vi "OPC Main.vi"(7 "Name of Parent Panel":string="Main.vi", 9 "New Center Coords":T2={"Horizontal"=470, "Vertical"=200}, 10 "Config":variant, 11 "Main UI Message Queue":refnum<queue>) -> ()   [LabVIEW 2018, in "OPC UA.lvlib"]
uses:
  OPC UA.lvlib
  support/Message Queue/Message Cluster.ctl
  <vilib>/Utility/miscctls.llb/LVPoint32TypeDef.ctl
  OPC Tag Data.ctl
  controls/UI State.ctl
  OPC Module Config.ctl
  Scale Module Folder/Measure Instrument/State Enum.ctl
  OPC Settings.ctl
  Variable Data Cluster.ctl
  <vilib>/OPCUA/controls/NodeId.ctl
  <vilib>/OPCUA/controls/OPC UA StatusCode.ctl
  <vilib>/OPCUA/controls/Subscription ID.ctl
  <vilib>/OPCUA/controls/OPC UA Client Refnum.ctl
  <vilib>/OPCUA/controls/Subscription Data Change.ctl
  <vilib>/OPCUA/controls/Data Type.ctl
  OPC Display Cluster.ctl
  support/Message Queue/Enqueue Message (Single).vi
  support/Message Queue/Message Queue.lvlib
  support/Support Library.lvlib
  support/Command Log VIs/Command Logging.lvlib
  support/User Event - Stop/User Event - Stop.lvlib
  OPC Dialog.vi
  Scale Module Folder/Measure Instrument/Scale Module Engine.lvlib
  OPC UA Module Engine.lvlib
  Report Generation/Report Generation.lvlib
panel:
  out "Tag Data 2":T1[](array[typedef])
  out "Configuration.server endpoint URL":string
  out "Updating":bool
  out "ScanCode":i16
  in  "Settings Button":bool
  in  "Exit":bool
  out "Status":string
  out "Log File path":path
  out "server endpoint URL":string
  # "opc.tcp://localhost:49580"
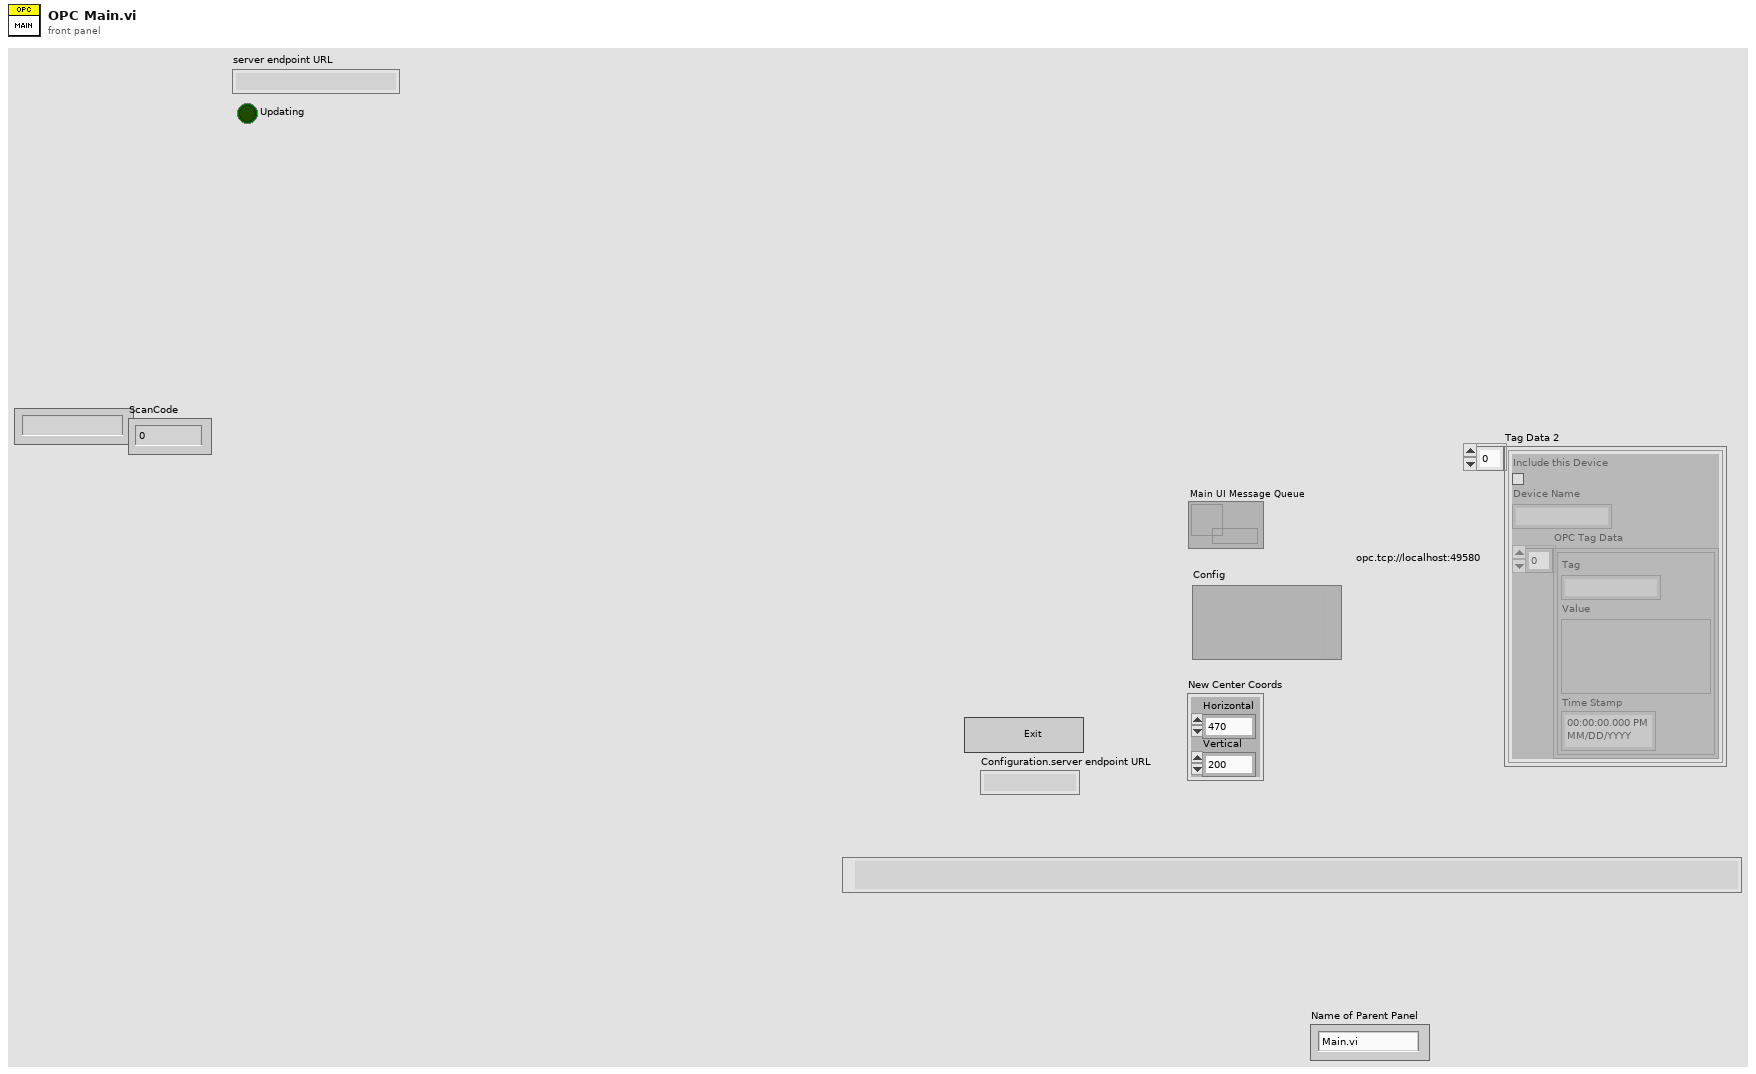
[diagram p1: front panel]
types:
  T1 = typedef "OPC UA.lvlib/OPC Tag Data.ctl" = cluster{"Include this Device":bool, "Device Name":string, "OPC Tag Data":cluster{"Tag":string, "Value":variant, "Time Stamp":timestamp}[]}
  T2 = typedef "LVPoint32TypeDef.ctl" = cluster{"Horizontal":i32, "Vertical":i32}
  T3 = enum32{"Invalid", "Default", "Floating", "Floating/Auto-Hide", "Modal"}
  T4 = typedef "OPC UA.lvlib/OPC Module Config.ctl" = cluster{"State":T5, "GUID":string, "Process Name":string, "User name":string, "Drop Coords":T2, "Configuration":T6, "First Iteration":bool, "Data":cluster{"Object Name":string, "Variable Array":T7[]}[], "Load Count":i32, "Log Started":bool, "subscription ID out":T10, "OPC UA client refnum out":T11, "Event Registration Refnum":refnum<event-registration>, "Start Time":timestamp, "Current Time":timestamp, "Tag Data":T1[]}
  T5 = typedef "Scale Module.lvlib/Scale Module Engine.lvlib/State Enum.ctl" = enum16{"Measuring", "Idle"}
  T6 = typedef "OPC UA.lvlib/OPC Settings.ctl" = cluster{"Cycle Period":dbl, "server endpoint URL":string, "security policy":cluster{"message mode":enum16{"None", "Sign", "Sign and Encrypt"}, "security":enum16{"Basic256", "Basic128Rsa15"}}, "Trust Any Server":bool}
  T7 = typedef "OPC UA.lvlib/Variable Data Cluster.ctl" = cluster{"node ID":T8, "browse name":string, "status":T9, "timestamp":timestamp, "value ":variant}
  T8 = typedef "NodeId.ctl" = string
  T9 = typedef "OPC UA StatusCode.ctl" = u32
  T10 = typedef "Subscription ID.ctl" = u32
  T11 = typedef "OPC UA Client Refnum.ctl" = refnum<k21>
  T12 = typedef "UI State.ctl" = enum16{"Idle", "Acquiring and Logging", "Waiting for Exit", "Waiting for Exit (Acq Stopped)", "Waiting for Exit (Log Stopped)", "Waiting for Stop", "Waiting for Stop (Acq Stopped)", "Waiting for Stop (Log Stopped)"}
  T13 = typedef "OPC UA.lvlib/Message Queues.ctl" = cluster{"OPC UI":refnum<queue>, "OPC Engine":refnum<queue>, "OPC Display":refnum<queue>}
  T14 = typedef "OPC UA.lvlib/OPC Display Cluster.ctl" = cluster{"URL":string, "Cycle":i32, "Updating":bool, "Tag Data":T1[]}
  T15 = cluster{"Shift":bool, "Ctrl":bool, "Alt":bool, "Cmd":bool, "Opt":bool}
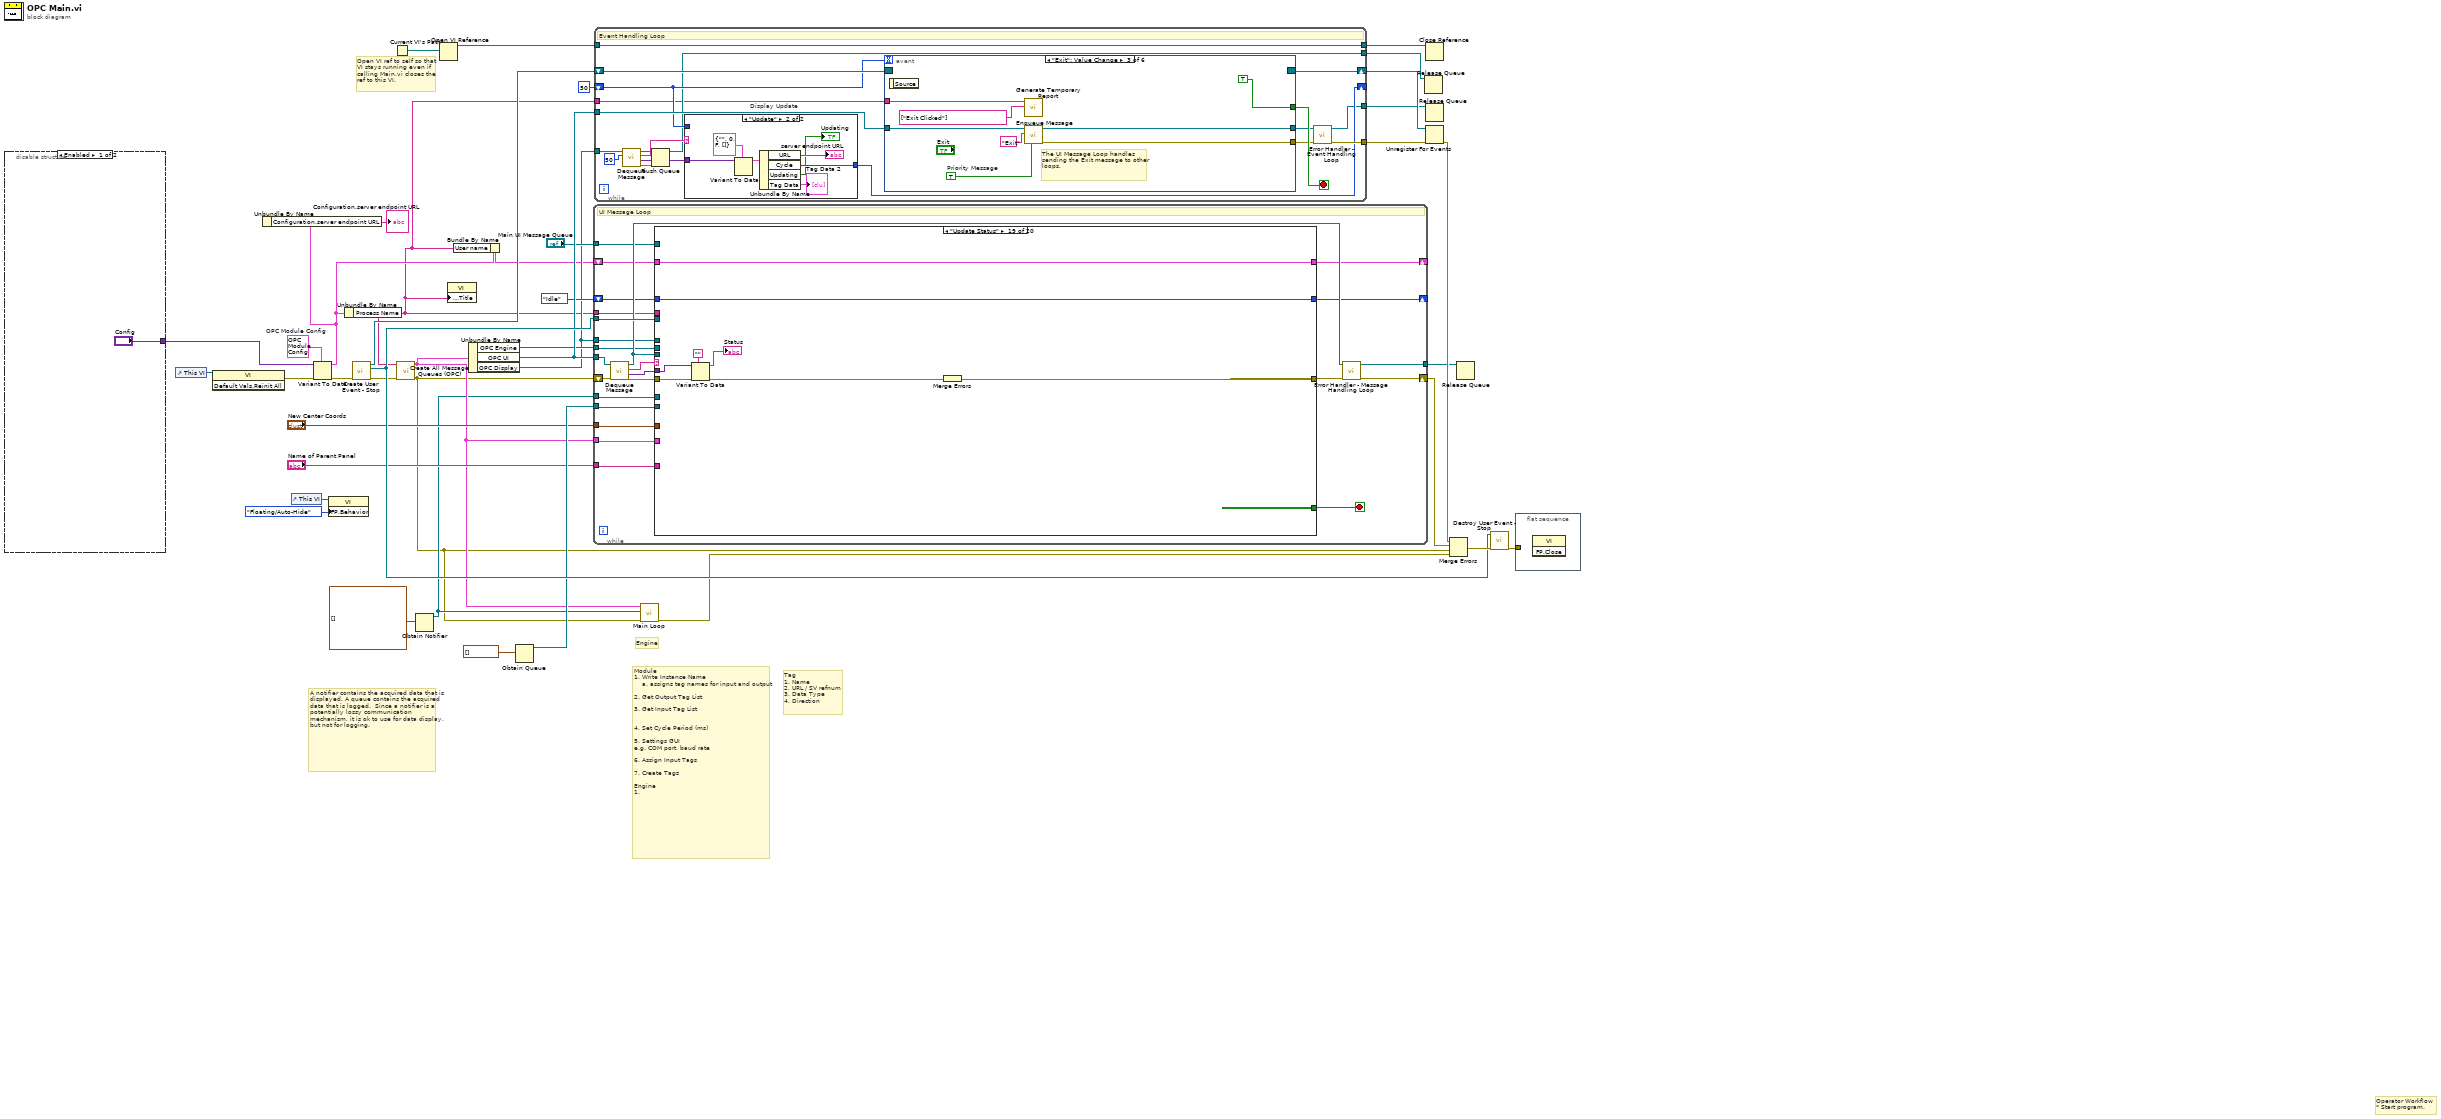
[diagram p0: block diagram]
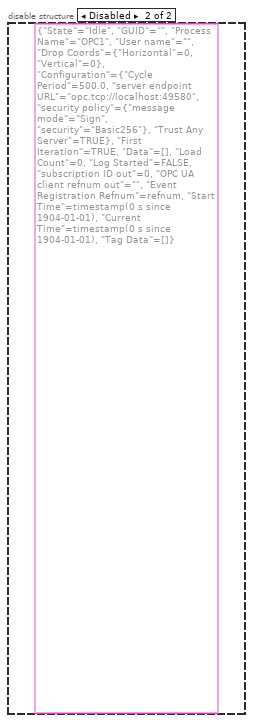
[diagram p2: hidden frame]
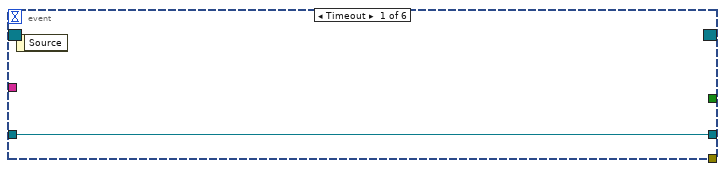
[diagram p4: hidden frame]
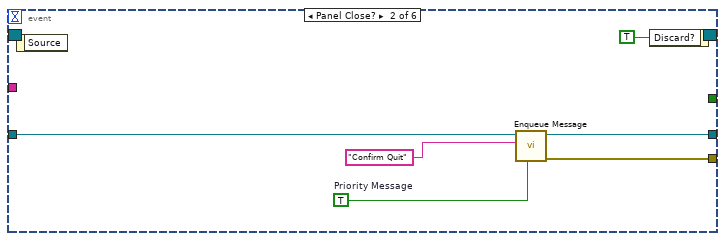
[diagram p5: hidden frame]
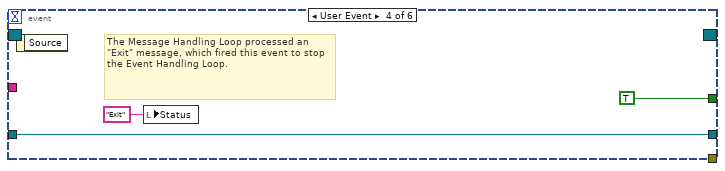
[diagram p6: hidden frame]
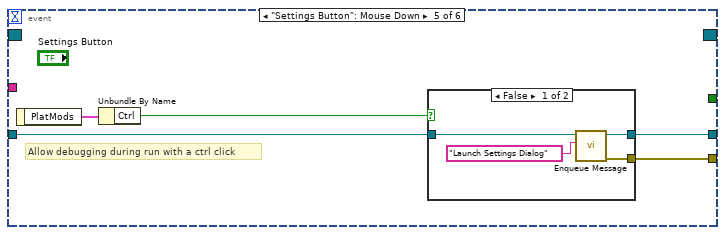
[diagram p7: hidden frame]
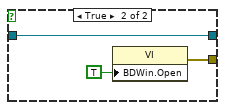
[diagram p8: hidden frame]
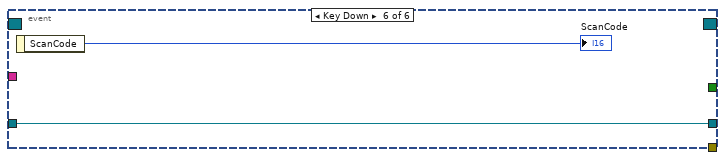
[diagram p9: hidden frame]
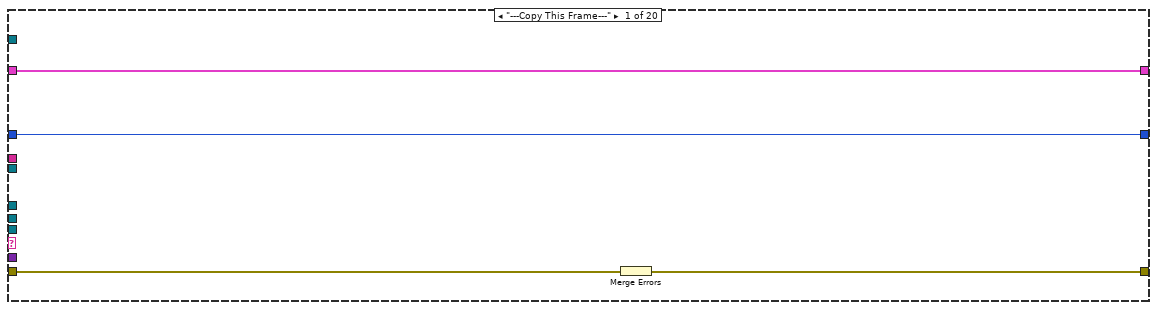
[diagram p10: hidden frame]
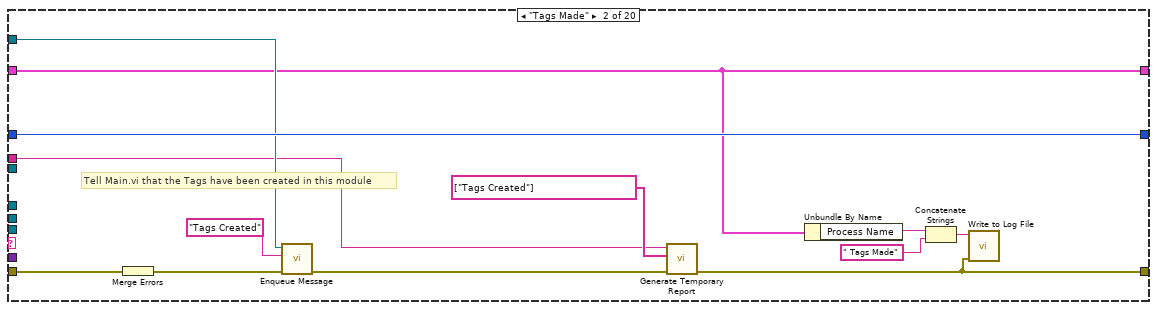
[diagram p11: hidden frame]
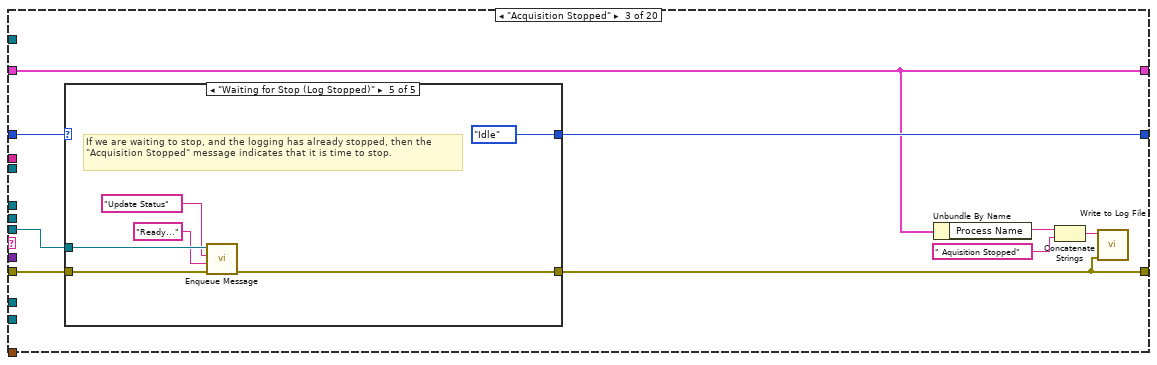
[diagram p12: hidden frame]
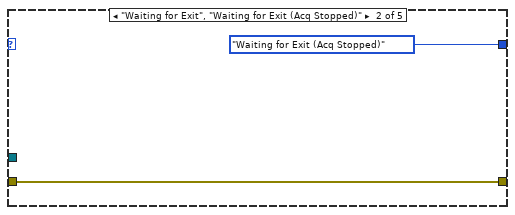
[diagram p14: hidden frame]
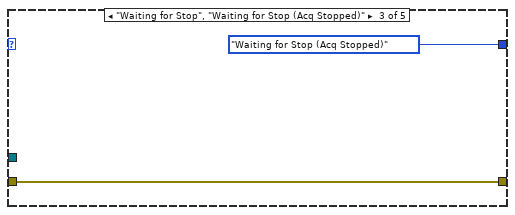
[diagram p15: hidden frame]
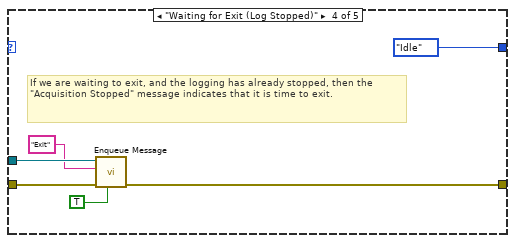
[diagram p16: hidden frame]
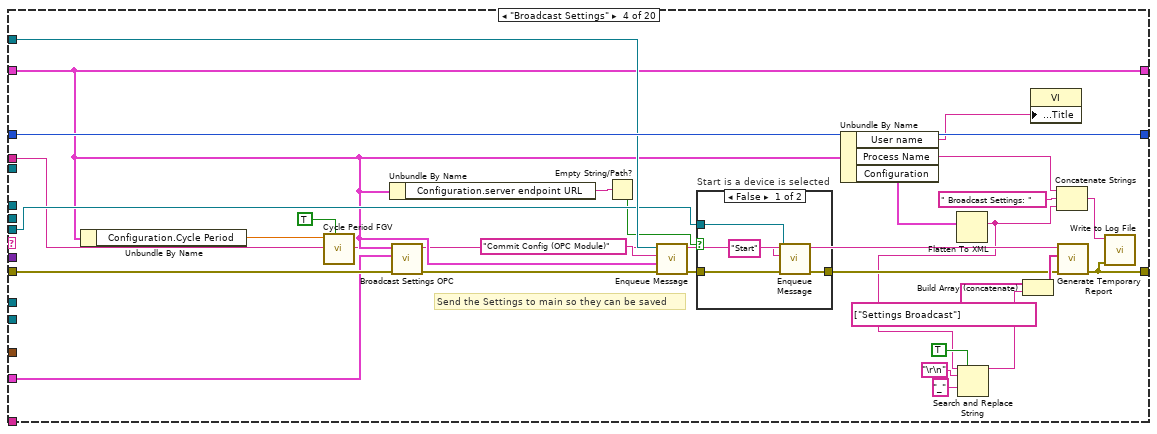
[diagram p17: hidden frame]
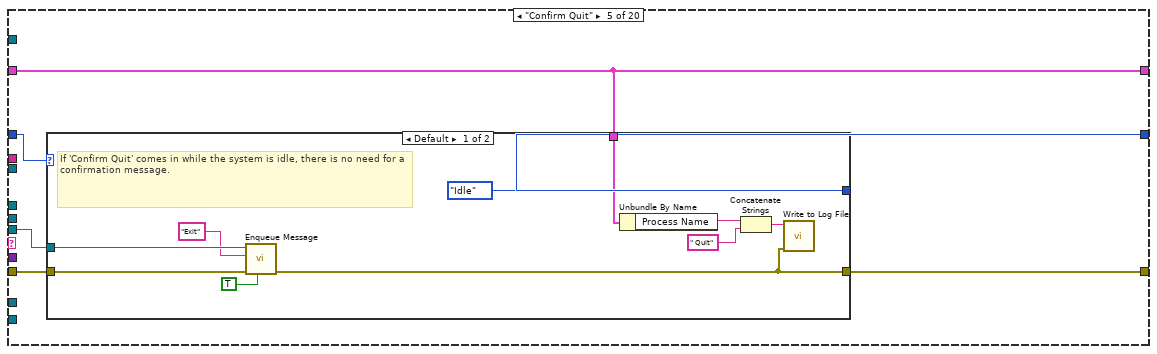
[diagram p19: hidden frame]
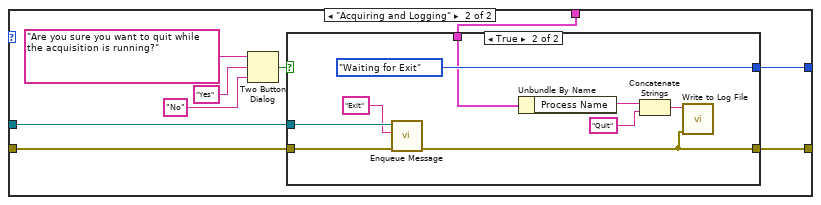
[diagram p20: hidden frame]
diagram:
  w7 = T4 {"State"=enum."Idle", "GUID"="", "Process Name"="", "User name"="", "Drop Coords"={"Horizontal"=0, "Vertical"=0}, "Configuration"={"Cycle Period"=500.0, "server endpoint URL"="", "security policy"={"message mode"=enum."Sign", "security"=enum."Basic256"}, "Trust Any Server"=FALSE}, "First Iteration"=FALSE, "Data"=[], "Load Count"=0, "Log Started"=FALSE, "subscription ID out"=0, "OPC UA client refnum out"="", "Event Registration Refnum"=refnum, "Start Time"=timestamp(0 s since 1904-01-01), "Current Time"=timestamp(0 s since 1904-01-01), "Tag Data"=[]}  # OPC Module Config
  # "Open VI ref to self so that\nVI stays running even if\ncalling Main.vi closes the\nref to this VI."
  # "Engine"
  # "Operator Workflow\n* Start program."
  # "Module \n1. Write Instance Name\n    a. assigns tag names for input and output\n\n2. Get Output Tag List\n\n3. Get Input Tag List\n\n\n4. Set Cycle Period (ms)\n\n5. Settings GUI\ne.g. COM port, baud rate\n\n6. Assign Input Tags\n\n7. Create Tags\n\nEngine\n1."
  # "Tag\n1. Name\n2. URL / SV refnum\n3. Data Type\n4. Direction"
  # "A notifier contains the acquired data that is displayed. A queue contains the acquired data that is logged.  Since a notifier is a potentially lossy communication mechanism, it is ok to use for data display, but not for logging."
  n1 = disable-structure shown="Enabled" {
    disable-tunnel: ["Config" _] -> w14
    frame Enabled {
    }
    frame Disabled {
      (unwired) T4 {"State"=enum."Idle", "GUID"="", "Process Name"="OPC1", "User name"="", "Drop Coords"={"Horizontal"=0, "Vertical"=0}, "Configuration"={"Cycle Period"=500.0, "server endpoint URL"="opc.tcp://localhost:49580", "security policy"={"message mode"=enum."Sign", "security"=enum."Basic256"}, "Trust Any Server"=TRUE}, "First Iteration"=TRUE, "Data"=[], "Load Count"=0, "Log Started"=FALSE, "subscription ID out"=0, "OPC UA client refnum out"="", "Event Registration Refnum"=refnum, "Start Time"=timestamp(0 s since 1904-01-01), "Current Time"=timestamp(0 s since 1904-01-01), "Tag Data"=[]} ("OPC Module Config")
    }
  }
  n2 = control-ref of="This VI"() -> (w6:refnum<vi>)
  n3 = invoke class="VI" method="Default Vals.Reinit All"(reference=w6) -> (error out=w20:errorcluster)  [unwired: 2 in, 2 out]
  n4 = control-ref of="This VI"() -> (w5:refnum<vi>)
  n5 = Variant To Data(error in=w20, type=w7, Variant=w14) -> (data=w3:T4, error out=w25:errorcluster)
  n6 = Unbundle By Name(w3) -> ("Configuration.server endpoint URL"=→"Configuration.server endpoint URL":string)
  n7 = property class="VI"(reference=w5, "FP.Behavior"=T3."Floating/Auto-Hide" ("Front Panel Window:Behavior")) -> ()  [unwired: 1 in, 2 out]
  n8 = Unbundle By Name(w3) -> ("Process Name"=w1:string)
  n9 = call "Create User Event - Stop.vi"("error in (no error)"=w25) -> ("error out"=w19:errorcluster, "User Event - Stop"=w37:refnum<user-event>, "Stop Event Registration Refnum"=w38:refnum<event-registration>)  [unwired: 8 in]
  n10 = Current VI's Path() -> (path=w26:path)
  n11 = call "Create All Message Queues (OPC).vi"("error in (no error)"=w19, "Process Name"=w1) -> ("error out"=w16:errorcluster, "Message Queues"=w18:T13)  [unwired: 8 in]
  n12 = Obtain Notifier(notification data type=waveform(dbl)[] []) -> (notifier out=w17:refnum<notifier>)  [unwired: 3 in, 2 out]
  n13 = Open VI Reference(vi path=w26) -> (vi reference=w27:refnum<vi>)  [unwired: 5 in, 1 out]
  n14 = property class="VI"("Front Panel.Title"=w1) -> ()  [unwired: 2 in, 2 out]
  n15 = Bundle By Name(cluster=w3, "User name"=w1) -> (w2:T4)
  n16 = Unbundle By Name(w18) -> ("OPC Engine"=w30:refnum<queue>, "OPC UI"=w34:refnum<queue>, "OPC Display"=w13:refnum<queue>)
  n17 = Obtain Queue(element data type=waveform(dbl)[] []) -> (queue out=w29:refnum<queue>)  [unwired: 4 in, 2 out]
  n18 = while {
    tunnel: w34 -> [w61]
    tunnel: w37 -> [w65]
    shift-right: [w57] -> w41
    shift-left: w16 -> [w64]
    shift-right: [w43] -> _
    shift-left: w2 -> [w50]
    tunnel: w17 -> [w60]
    tunnel: w29 -> [w59]
    shift-right: [w54] -> _
    shift-left: UI_State."Idle" ("UI State") -> [w55]
    tunnel: w30 -> [w53]
    tunnel: w18 -> [w52]
    tunnel: "Main UI Message Queue" -> [w49]
    tunnel: w1 -> [w48]
    tunnel: "New Center Coords" -> [w47]
    tunnel: "Name of Parent Panel" -> [w46]
    tunnel: w13 -> [w45]
    tunnel: [w44] -> w8
    stop <- w66 stop-if-true
    # "UI Message Loop"
    n19 = call "Dequeue Message.vi"("error in (no error)"=w64, "Message Queue"=w61) -> ("error out"=w51:errorcluster, "Message Data"=w62:variant, "Message"=w63:string, "dup Message Queue"=w56:refnum<queue>)  [unwired: 6 in]
    n20 = case "Message Cases" shown="\"Update Status\"" w63 {
      selector: w63 -> [_ _ _ _ _ _ _ _ _ _ _ _ _ _ _ _ _ _ _ w417]
      tunnel: w56 -> [_ _ w89 w133 w148 _ w201 w215 w239 _ w281 w298 w314 _ w352 _ _ w405 _ _]
      tunnel: w51 -> [w70 w83 w90 w126 w147 w182 w196 w219 w238 w264 w277 w293 w315 w338 w351 w360 w372 w400 w414 _]
      tunnel: [w69 w71 w85 w116 w146 w183 w188 w206 w221 w264 w265 w288 w310 w341 w346 w357 w374 w388 w415 w416] -> w58
      tunnel: [_ _ _ _ _ _ _ _ TRUE _ _ _ _ _ _ _ _ _ _ _] -> w66
      tunnel: w62 -> [_ _ _ _ _ w185 _ w218 w228 _ _ _ _ w339 _ _ _ _ w413 _]
      tunnel: w65 -> [_ _ _ _ _ _ _ _ w249 _ _ _ _ _ _ _ _ _ _ _]
      tunnel: w50 -> [w67 w75 w84 w123 w144 w180 w191 w205 w224 w261 w269 w291 w309 w345 w347 w361 w373 w392 w408 w422]
      tunnel: w60 -> [_ _ _ _ _ _ _ _ w247 _ _ _ _ _ _ _ _ _ _ _]
      tunnel: w59 -> [_ _ _ _ _ _ _ _ w243 _ _ _ _ _ _ _ _ _ _ _]
      tunnel: w55 -> [w68 w82 w92 w138 w149 w181 w197 w210 w236 _ _ w300 w317 w344 _ _ _ w401 w409 w426]
      tunnel: [w68 w82 w91 w138 w145 w181 w198 w210 w235 UI_State."Idle" ("UI State") UI_State."Idle" ("UI State") w300 w316 w344 UI_State."Acquiring and Logging" ("UI State") UI_State."Acquiring and Logging" ("UI State") UI_State."Acquiring and Logging" ("UI State") w402 w409 w426] -> w54
      tunnel: w53 -> [_ _ _ _ _ _ _ _ w242 _ _ _ _ _ _ w365 w381 w399 _ _]
      tunnel: w52 -> [_ _ _ w124 _ _ _ _ _ _ _ _ _ _ _ _ _ _ _ _]
      tunnel: w49 -> [_ w79 _ w134 _ _ _ _ w227 _ _ w299 _ _ _ _ _ _ _ _]
      tunnel: [w67 w75 w84 w123 w144 w180 w191 w205 w224 w261 w269 w292 w309 w345 w347 w361 w373 w392 w408 w422] -> w43
      tunnel: w48 -> [_ w73 _ w118 _ _ w187 _ _ _ w275 _ _ _ _ w356 _ w390 _ _]
      tunnel: w47 -> [_ _ _ _ _ _ _ _ _ _ w274 _ _ _ _ _ _ _ _ _]
      tunnel: w46 -> [_ _ _ _ _ _ _ _ _ _ w273 _ _ _ _ _ _ _ _ _]
      tunnel: w45 -> [_ _ _ _ _ _ _ _ _ _ w268 _ _ _ _ _ _ _ _ _]
      frame "---Copy This Frame---" {
        # "Duplicate this frame when creating new messages.  Change this comment in the duplicated frame to describe this message."
        n21 = Merge Errors(w70) -> (w69:errorcluster)
      }
      frame "Tags Made" {
        # "Tell Main.vi that the Tags have been created in this module"
        # "Duplicate this frame when creating new messages.  Change this comment in the duplicated frame to describe this message."
        n22 = Merge Errors(w83) -> (w80:errorcluster)
        n23 = call-poly "Enqueue Message.vi"("error in (no error)"=w80, "Message"="Tags Created", "Message Queue"=w79) -> ("error out"=w72:errorcluster)  [unwired: 7 in, 1 out]
        n24 = call "Generate Temporary Report.vi"("error in (no error)"=w72, "Line of Events"=string[] ["Tags Created"], "Module Name"=w73) -> ("error out"=w71:errorcluster)  [unwired: 8 in]
        n25 = Unbundle By Name(w75) -> ("Process Name"=w78:string)
        n26 = Concatenate Strings(w78, " Tags Made" ("text")) -> (w76:string)
        n27 = call "Write to Log File.vi"("error in"=w71, "text"=w76) -> ()  [unwired: 9 in, 1 out]
      }
      frame "Acquisition Stopped" {
        # "Logic for determining what action to take when the acquisition has stopped."
        n28 = case shown="\"Waiting for Stop (Log Stopped)\"" w92 {
          selector: w92 -> [w94 _ _ _ _]
          tunnel: [w94 UI_State."Waiting for Exit (Acq Stopped)" ("UI State") UI_State."Waiting for Stop (Acq Stopped)" ("UI State") UI_State."Idle" ("UI State") UI_State."Idle" ("UI State")] -> w91
          tunnel: w90 -> [w93 w95 w97 w103 w109]
          tunnel: [w93 w95 w97 w102 w108] -> w85
          tunnel: w89 -> [_ _ _ w101 w107]
          frame Default {
          }
          frame "Waiting for Exit", "Waiting for Exit (Acq Stopped)" {
          }
          frame "Waiting for Stop", "Waiting for Stop (Acq Stopped)" {
          }
          frame "Waiting for Exit (Log Stopped)" {
            # "If we are waiting to exit, and the logging has already stopped, then the \"Acquisition Stopped\" message indicates that it is time to exit."
            n29 = call-poly "Enqueue Message.vi"("Priority Message? (F)"=TRUE, "error in (no error)"=w103, "Message"="Exit", "Message Queue"=w101) -> ("error out"=w102:errorcluster)  [unwired: 6 in, 1 out]
          }
          frame "Waiting for Stop (Log Stopped)" {
            # "If we are waiting to stop, and the logging has already stopped, then the \"Acquisition Stopped\" message indicates that it is time to stop."
            n30 = call-poly "Enqueue Message.vi"("error in (no error)"=w109, "Message Data"="Ready..." ("Message"), "Message"="Update Status", "Message Queue"=w107) -> ("error out"=w108:errorcluster)  [unwired: 6 in, 1 out]
          }
        }
        n31 = Unbundle By Name(w84) -> ("Process Name"=w88:string)
        n32 = Concatenate Strings(w88, " Aquisition Stopped" ("text")) -> (w86:string)
        n33 = call "Write to Log File.vi"("error in"=w85, "text"=w86) -> ()  [unwired: 9 in, 1 out]
      }
      frame "Broadcast Settings" {
        # "Send the Settings to main so they can be saved"
        # "Send the 'Update Settings' message to the Logging and Acquisition message loops."
        n34 = Unbundle By Name(w123) -> ("Configuration.Cycle Period"=w136:dbl)
        n35 = call "Cycle Period FGV.vi"("Write"=TRUE, "Cycle Period In (ms)"=w136) -> ()  [unwired: 8 in, 2 out]
        n36 = Unbundle By Name(w123) -> ("Configuration.server endpoint URL"=w128:string)
        n37 = call "Broadcast Settings OPC.vi"("error in (no error)"=w126, "Message Queues"=w124, "OPC Module Config"=w123) -> ("error out"=w125:errorcluster)  [unwired: 8 in]
        n38 = Empty String/Path?(string/path=w128) -> (empty?=w127:bool)
        n39 = call-poly "Enqueue Message.vi"("error in (no error)"=w125, "Message Data"=w123, "Message"="Commit Config (OPC Module)", "Message Queue"=w134) -> ("error out"=w132:errorcluster)  [unwired: 6 in, 1 out]
        n40 = case "Start is a device is selected" shown="False" w127 {
          tunnel: w133 -> [w141 _]
          tunnel: w132 -> [w140 w143]
          tunnel: [w139 w143] -> w117
          frame False {
            n41 = call-poly "Enqueue Message.vi"("error in (no error)"=w140, "Message"="Start", "Message Queue"=w141) -> ("error out"=w139:errorcluster)  [unwired: 7 in, 1 out]
          }
          frame True {
          }
        }
        n42 = Unbundle By Name(w123) -> ("User name"=w121:string, "Process Name"=w122:string, "Configuration"=w129:T6)
        n43 = Flatten To XML(anything=w129) -> (xml string=w112:string)
        n44 = Search and Replace String(replace all?=TRUE ("replace all? (F)"), input string=w112, search string="\r\n", replace string="_" ("replace string (\"\")")) -> (result string=w111:string)  [unwired: 4 in, 3 out]
        n45 = Build Array (concatenate)(string[] ["Settings Broadcast"] ("Line of Events"), w111) -> (w119:string[])
        n46 = property class="VI"("Front Panel.Title"=w121) -> ()  [unwired: 2 in, 2 out]
        n47 = Concatenate Strings(w122, " Broadcast Settings: " ("text"), w112) -> (w130:string)
        n48 = call "Generate Temporary Report.vi"("error in (no error)"=w117, "Line of Events"=w119, "Module Name"=w118) -> ("error out"=w116:errorcluster)  [unwired: 8 in]
        n49 = call "Write to Log File.vi"("error in"=w116, "text"=w130) -> ()  [unwired: 9 in, 1 out]
      }
      frame "Confirm Quit" {
        # "Confirm Quit - Message that can confirm whether or not the user wants to exit the application."
        n50 = case shown="Default" w149 {
          tunnel: w148 -> [w158 w165]
          tunnel: w147 -> [w157 w163]
          tunnel: [w151 w162] -> w146
          tunnel: [UI_State."Idle" ("UI State") w161] -> w145
          tunnel: w144 -> [w150 w160]
          frame Default {
            # "If 'Confirm Quit' comes in while the system is idle, there is no need for a confirmation message."
            n51 = call-poly "Enqueue Message.vi"("Priority Message? (F)"=TRUE, "error in (no error)"=w157, "Message"="Exit", "Message Queue"=w158) -> ("error out"=w151:errorcluster)  [unwired: 6 in, 1 out]
            n52 = Unbundle By Name(w150) -> ("Process Name"=w154:string)
            n53 = Concatenate Strings(w154, " Quit" ("text")) -> (w152:string)
            n54 = call "Write to Log File.vi"("error in"=w151, "text"=w152) -> ()  [unwired: 9 in, 1 out]
          }
          frame "Acquiring and Logging" {
            n55 = Two Button Dialog(message="Are you sure you want to quit while the acquisition is running?" ("Confirm Quit Message"), 1:"No" ("No"), 2:"Yes" ("Yes")) -> (T button?=w164:bool)
            n56 = case shown="True" w164 {
              tunnel: w165 -> [_ w179]
              tunnel: w163 -> [w169 w178]
              tunnel: [w169 w172] -> w162
              tunnel: [UI_State."Acquiring and Logging" ("UI State") UI_State."Waiting for Exit" ("UI State")] -> w161
              tunnel: w160 -> [_ w171]
              frame False {
                # "User did not want to quit."
              }
              frame True {
                n57 = call-poly "Enqueue Message.vi"("error in (no error)"=w178, "Message"="Exit", "Message Queue"=w179) -> ("error out"=w172:errorcluster)  [unwired: 7 in, 1 out]
                n58 = Unbundle By Name(w171) -> ("Process Name"=w175:string)
                n59 = Concatenate Strings(w175, "Quit" ("text")) -> (w173:string)
                n60 = call "Write to Log File.vi"("error in"=w172, "text"=w173) -> ()  [unwired: 9 in, 1 out]
              }
            }
          }
        }
      }
      frame "Display Log File Path" {
        n61 = Variant To Data(error in=w182, type=path "", Variant=w185) -> (data=→"Log File path":path, error out=w183:errorcluster)
      }
      frame "E-Stop" {
        # "E-Stop has no effect on the scale"
        # "Message Acquisition and Logging loops to stop"
        # "Stop the pumps."
        n62 = call-poly "Enqueue Message.vi"("error in (no error)"=w196, "Message Data"="Ready..." ("Ready..."), "Message"="Update Status", "Message Queue"=w201) -> ("error out"=w195:errorcluster)  [unwired: 6 in, 1 out]
        n63 = case shown="\"Waiting for Exit\"" w197 {
          selector: w197 -> [_ w203]
          tunnel: [UI_State."Waiting for Stop" ("UI State") w203] -> w198
          frame Default {
          }
          frame "Waiting for Exit" {
          }
        }
        n64 = Merge Errors(w195) -> (w189:errorcluster)
        n65 = Unbundle By Name(w191) -> ("Process Name"=w194:string)
        n66 = call "Generate Temporary Report.vi"("error in (no error)"=w189, "Line of Events"=string[] ["E-STOP"], "Module Name"=w187) -> ("error out"=w188:errorcluster)  [unwired: 8 in]
        n67 = Concatenate Strings(w194, " E-STOP" ("text")) -> (w192:string)
        n68 = call "Write to Log File.vi"("error in"=w188, "text"=w192) -> ()  [unwired: 9 in, 1 out]
      }
      frame "Error" {
        # "Error - Check the error message data and respond accordingly. This message is sent by the \"Error Handler\" VIs at the end of each loop in this application."
        n69 = Variant To Data(error in=w219, type=errorcluster {"status"=FALSE, "code"=0, "source"=""} ("error out"), Variant=w218) -> (data=w216:errorcluster, error out=w212:errorcluster)
        n70 = call <vilib>:"General Error Handler.vi"("error in (no error)"=w216) -> ("message"=w204:string)  [unwired: 10 in, 4 out]
        n71 = call-poly "Enqueue Message.vi"("Priority Message? (F)"=TRUE, "Message"="Exit", "Message Queue"=w215) -> ("error out"=w211:errorcluster)  [unwired: 7 in, 1 out]
        n72 = Merge Errors(w211, w212) -> (w206:errorcluster)
        n73 = Unbundle By Name(w205) -> ("Process Name"=w209:string)
        n74 = Concatenate Strings(w209, " Error: " ("text"), w204) -> (w207:string)
        n75 = call "Write to Log File.vi"("error in"=w206, "text"=w207) -> ()  [unwired: 9 in, 1 out]
      }
      frame "Exit" {
        w231 = TRUE  # Delete Module?
        # "Don't check the error outs. The acquisition and logging queues may have already been released."
        # "Close references owned by the Main VI."
        # "Stop the VI"
        # "Exit - Fire the User Event to stop the Event Handling Loop.  Also send Exit messages to the Acquisition and Logging loops."
        n76 = call "Fire User Event - Stop.vi"("User Event - Stop"=w249) -> ("error out"=w248:errorcluster)  [unwired: 10 in]
        n77 = Build Array(w242) -> (w241:refnum<queue>[])
        n78 = for {
          tunnel: w241 -> [w258] mode=indexing
          n79 = call-poly "Enqueue Message.vi"("Message"="Stop", "Message Queue"=w258) -> ("dup Message Queue"=w259:refnum<queue>)  [unwired: 8 in, 1 out]
          n80 = call-poly "Enqueue Message.vi"("Message"="Exit", "Message Queue"=w259) -> ()  [unwired: 8 in, 2 out]
        }
        n81 = Variant To Data(type=w231, Variant=w228) -> (data=w230:bool, error out=w232:errorcluster)  [unwired: 1 in]
        n82 = call-poly "Enqueue Message.vi"("error in (no error)"=w238, "Message Data"="Ready..." ("Ready..."), "Message"="Update Status", "Message Queue"=w239) -> ("error out"=w237:errorcluster, "dup Message Queue"=w234:refnum<queue>)  [unwired: 6 in]
        n83 = Select(t=w231, s=w232, f=w230) -> (s? t:f=w229:bool)
        n84 = case "Don't enqueue Delete Module if opening campaign because it\nwill already have been deleted and new config loaded and we create\na race condition." shown="True" w229 {
          tunnel: w227 -> [_ w253]
          tunnel: w224 -> [_ w252]
          frame False {
          }
          frame True {
            n85 = Unbundle By Name(w252) -> ("GUID"=w251:string)
            n86 = call-poly "Enqueue Message.vi"("Message Data"=w251, "Message"="Delete Module", "Message Queue"=w253) -> ()  [unwired: 7 in, 2 out]
          }
        }
        n87 = Release Queue(queue=w234, error in (no error)=w237) -> (error out=w246:errorcluster)  [unwired: 1 in, 2 out]
        n88 = Release Notifier(notifier=w247, error in (no error)=w246) -> (error out=w245:errorcluster)  [unwired: 1 in, 2 out]
        n89 = Release Queue(queue=w243, error in (no error)=w245) -> (error out=w244:errorcluster)  [unwired: 1 in, 2 out]
        n90 = Merge Errors(w248, w244) -> (w222:errorcluster)
        n91 = case shown="Default" w236 {
          selector: w236 -> [_ w256]
          tunnel: [UI_State."Waiting for Stop" ("UI State") w256] -> w235
          frame Default {
          }
          frame "Waiting for Exit" {
          }
        }
        n92 = Unbundle By Name(w224) -> ("Process Name"=w220:string)
        n93 = call "Generate Temporary Report.vi"("error in (no error)"=w222, "Line of Events"=string[] ["Exited"], "Module Name"=w220) -> ("error out"=w221:errorcluster)  [unwired: 8 in]
        n94 = Concatenate Strings(w220, " Exit" ("text")) -> (w225:string)
        n95 = call "Write to Log File.vi"("error in"=w221, "text"=w225) -> ()  [unwired: 9 in, 1 out]
      }
      frame "Init UI Refs" {
        # "Init UI Refs - Store control references for UI controls.  Also enable/disable controls appropriately."
        n96 = property class="VI"("Front Panel.Closeable"=TRUE ("Front Panel Window:Closeable")) -> ()  [unwired: 2 in, 2 out]
      }
      frame "Initialize" {
        # "Initialize - Get configuration settings, then message the UI to initialize, and broadcast the settings to the other message loops."
        n97 = call-poly "Enqueue Message.vi"("error in (no error)"=w277, "Message"="Init UI Refs", "Message Queue"=w281) -> ("error out"=w279:errorcluster, "dup Message Queue"=w280:refnum<queue>)  [unwired: 7 in]
        n98 = property class="VI" props=["FP.State"]() -> (reference out=w276:refnum<vi>)  [unwired: 2 in, 2 out]
        n99 = call "Make Child and Move.vi"("Process Name"=w275, "Name of Parent Panel"=w273, "New Center Coords"=w274, "VI in"=w276) -> ()  [unwired: 8 in]
        n100 = call-poly "Enqueue Message.vi"("error in (no error)"=w279, "Message"="Broadcast Settings", "Message Queue"=w280) -> ("error out"=w287:errorcluster, "dup Message Queue"=w286:refnum<queue>)  [unwired: 7 in]
        n101 = call-poly "Enqueue Message.vi"("error in (no error)"=w287, "Message Data"="Ready..." ("Ready..."), "Message"="Update Status", "Message Queue"=w286) -> ("error out"=w266:errorcluster)  [unwired: 6 in, 1 out]
        n102 = call "Update if Clear.vi"("error in (no error)"=w266, "Message Data"=T14 {"URL"="", "Cycle"=0, "Updating"=FALSE, "Tag Data"=[]} ("OPC Display Cluster"), "Queue in"=w268) -> ("error out"=w265:errorcluster)  [unwired: 8 in]
        n103 = Unbundle By Name(w269) -> ("Process Name"=w272:string)
        n104 = Concatenate Strings(w272, " Initialize" ("text")) -> (w270:string)
        n105 = call "Write to Log File.vi"("error in"=w265, "text"=w270) -> ()  [unwired: 9 in, 1 out]
      }
      frame "Launch Settings Dialog" {
        # "Launch the Settings Dialog when the user clicks the 'Settings' button."
        n106 = in-place {
          n107 = in-place-cluster #1(w291) -> ("Load Count"=w301:i32)
          n108 = Increment(x=w301) -> (x+1=w302:i32)
          n109 = in-place-cluster #1("Load Count"=w302) -> (w290:T4)
        }
        n110 = call-by-ref "?"("error in (no error)"=w293, "OPC Module Config In"=w290) -> ("error out"=w289:errorcluster, "Cancelled?"=w294:bool, "OPC Module Config Out"=w292:T4)  [unwired: 8 in, 3 out]
        n111 = case shown="False" w294 {
          tunnel: w289 -> [w305 w308]
          tunnel: [w304 w308] -> w288
          tunnel: w299 -> [_ _]
          tunnel: w298 -> [w307 _]
          tunnel: w292 -> [w303 _]
          frame False {
            n112 = call-poly "Enqueue Message.vi"("error in (no error)"=w305, "Message Data"=w303, "Message"="Broadcast Settings", "Message Queue"=w307) -> ("error out"=w304:errorcluster)  [unwired: 6 in, 1 out]
          }
          frame True {
          }
        }
        n113 = Unbundle By Name(w292) -> ("Process Name"=w297:string)
        n114 = Concatenate Strings(w297, " Setting Dialog Launched" ("text")) -> (w295:string)
        n115 = call "Write to Log File.vi"("error in"=w288, "text"=w295) -> ()  [unwired: 9 in, 1 out]
      }
      frame "Logging Stopped" {
        # "Logic for determining what action to take when the logging has stopped."
        n116 = case shown="\"Waiting for Stop (Acq Stopped)\"" w317 {
          selector: w317 -> [w319 _ _ _ _]
          tunnel: [w319 UI_State."Waiting for Exit (Log Stopped)" ("UI State") UI_State."Waiting for Stop (Log Stopped)" ("UI State") UI_State."Idle" ("UI State") UI_State."Idle" ("UI State")] -> w316
          tunnel: w315 -> [w318 w320 w322 w328 w334]
          tunnel: [w318 w320 w322 w327 w333] -> w310
          tunnel: w314 -> [_ _ _ w326 w332]
          frame Default {
          }
          frame "Waiting for Exit", "Waiting for Exit (Log Stopped)" {
          }
          frame "Waiting for Stop", "Waiting for Stop (Log Stopped)" {
          }
          frame "Waiting for Exit (Acq Stopped)" {
            # "If we are waiting to exit, and the acquisition has already stopped, then the \"Logging Stopped\" message indicates that it is time to exit."
            n117 = call-poly "Enqueue Message.vi"("Priority Message? (F)"=TRUE, "error in (no error)"=w328, "Message"="Exit", "Message Queue"=w326) -> ("error out"=w327:errorcluster)  [unwired: 6 in, 1 out]
          }
          frame "Waiting for Stop (Acq Stopped)" {
            # "If we are waiting to stop, and the acquisition has already stopped, then the \"Logging Stopped\" message indicates that it is time to stop."
            n118 = call-poly "Enqueue Message.vi"("error in (no error)"=w334, "Message Data"="Ready..." ("Message"), "Message"="Update Status", "Message Queue"=w332) -> ("error out"=w333:errorcluster)  [unwired: 6 in, 1 out]
          }
        }
        n119 = Unbundle By Name(w309) -> ("Process Name"=w313:string)
        n120 = Concatenate Strings(w313, " Logging Stopped" ("text")) -> (w311:string)
        n121 = call "Write to Log File.vi"("error in"=w310, "text"=w311) -> ()  [unwired: 9 in, 1 out]
      }
      frame "Send to Sequencer" {
        n122 = Variant To Data(error in=w338, type=refnum<queue> refnum ("Message Queue"), Variant=w339) -> (data=w336:refnum<queue>, error out=w337:errorcluster)
        n123 = local read "Status"() -> (w342:string)
        n124 = call-poly "Enqueue Message.vi"("error in (no error)"=w337, "Message Data"=w342, "Message"="Sent to Sequence", "Message Queue"=w336) -> ("error out"=w341:errorcluster)  [unwired: 6 in, 1 out]
      }
      frame "Start" {
        # "Message Acquisition and Logging loops to start"
        # "Start - Enable/Disable buttons appropriately for an acquisition that has started, and update status display."
        n125 = call-poly "Enqueue Message.vi"("error in (no error)"=w351, "Message"="Start Loops", "Message Queue"=w352) -> ("error out"=w353:errorcluster)  [unwired: 7 in, 1 out]
        n126 = Merge Errors(w353) -> (w346:errorcluster)
        n127 = Unbundle By Name(w347) -> ("Process Name"=w350:string)
        n128 = Concatenate Strings(w350, " Start" ("text")) -> (w348:string)
        n129 = call "Write to Log File.vi"("error in"=w346, "text"=w348) -> ()  [unwired: 9 in, 1 out]
      }
      frame "Start Loops" {
        # "I'm not sure what we would have multiple Process names in a module for but i'll leave it for now."
        # "Message Acquisition and Logging loops to start"
        # "Start - Enable/Disable buttons appropriately for an acquisition that has started, and update status display."
        n130 = Build Array(w365) -> (w363:refnum<queue>[])
        n131 = Unbundle By Name(w361) -> ("Process Name"=w362:string)
        n132 = for {
          tunnel: w360 -> [w370]
          tunnel: [w369] -> w364 mode=indexing
          tunnel: w363 -> [w368] mode=indexing
          tunnel: w362 -> [w367]
          n133 = call-poly "Enqueue Message.vi"("error in (no error)"=w370, "Message Data"=w367, "Message"="Start", "Message Queue"=w368) -> ("error out"=w369:errorcluster)  [unwired: 6 in, 1 out]
        }
        n134 = Merge Errors(w360, w364) -> (w358:errorcluster)
        n135 = call "Generate Temporary Report.vi"("error in (no error)"=w358, "Line of Events"=string[] ["Started"], "Module Name"=w356) -> ("error out"=w357:errorcluster)  [unwired: 8 in]
      }
      frame "Start Log" {
        # "I'm not sure what we would have multiple Process names in a module for but i'll leave it for now."
        # "Message Acquisition and Logging loops to start"
        # "Start - Enable/Disable buttons appropriately for an acquisition that has started, and update status display."
        n136 = Build Array(w381) -> (w379:refnum<queue>[])
        n137 = Unbundle By Name(w373) -> ("Process Name"=w378:string)
        n138 = property class="VI"("Front Panel.Title"=w378) -> ()  [unwired: 2 in, 2 out]
        n139 = for {
          tunnel: w372 -> [w386]
          tunnel: [w385] -> w380 mode=indexing
          tunnel: w379 -> [w384] mode=indexing
          tunnel: w378 -> [w383]
          n140 = call-poly "Enqueue Message.vi"("error in (no error)"=w386, "Message Data"=w383, "Message"="Start Log", "Message Queue"=w384) -> ("error out"=w385:errorcluster)  [unwired: 6 in, 1 out]
        }
        n141 = Merge Errors(w372, w380) -> (w374:errorcluster)
        n142 = Unbundle By Name(w373) -> ("Process Name"=w377:string)
        n143 = Concatenate Strings(w377, " Start Log" ("text")) -> (w375:string)
        n144 = call "Write to Log File.vi"("error in"=w374, "text"=w375) -> ()  [unwired: 9 in, 1 out]
      }
      frame "Stop" {
        # "Stop - Enable/Disable buttons appropriately for an acquisition that has stopped, and update status display."
        n145 = call-poly "Enqueue Message.vi"("error in (no error)"=w400, "Message Data"="Ready..." ("Ready..."), "Message"="Update Status", "Message Queue"=w405) -> ("error out"=w398:errorcluster)  [unwired: 6 in, 1 out]
        n146 = call-poly "Enqueue Message.vi"("error in (no error)"=w398, "Message"="Stop", "Message Queue"=w399) -> ("error out"=w396:errorcluster)  [unwired: 7 in, 1 out]
        n147 = case shown="Default" w401 {
          selector: w401 -> [_ w407]
          tunnel: [UI_State."Waiting for Stop" ("UI State") w407] -> w402
          frame Default {
          }
          frame "Waiting for Exit" {
          }
        }
        n148 = Merge Errors(w396) -> (w389:errorcluster)
        n149 = Unbundle By Name(w392) -> ("Process Name"=w395:string)
        n150 = call "Generate Temporary Report.vi"("error in (no error)"=w389, "Line of Events"=string[] ["Stopped"], "Module Name"=w390) -> ("error out"=w388:errorcluster)  [unwired: 8 in]
        n151 = Concatenate Strings(w395, " Stop" ("text")) -> (w393:string)
        n152 = call "Write to Log File.vi"("error in"=w388, "text"=w393) -> ()  [unwired: 9 in, 1 out]
      }
      frame "Update Status" {
        # "Update Display - Convert the message data to a string to display in the Status indicator."
        n153 = Variant To Data(error in=w414, type="", Variant=w413) -> (data=→"Status":string, error out=w411:errorcluster)
        n154 = Merge Errors(w411) -> (w415:errorcluster)
      }
      frame Default {
        # "'Default' case only runs if there is a message that isn't defined in any of the other cases.  Output a programming error."
        n155 = Concatenate Strings("The invalid message string " ("string"), w417, " was received in OPC UA Main." ("string")) -> (w418:string)
        n156 = Bundle By Name(cluster=errorcluster {"status"=TRUE, "code"=1, "source"=""} ("error constant"), "source"=w418) -> (w416:errorcluster)
        n157 = Unbundle By Name(w422) -> ("Process Name"=w425:string)
        n158 = Concatenate Strings(w425, "Invalid Message Recieved" ("text"), w417) -> (w423:string)
        n159 = call "Write to Log File.vi"("text"=w423) -> ()  [unwired: 10 in, 1 out]
      }
    }
    n160 = call "Error Handler - Message Handling Loop.vi"("error in (no error)"=w58, "Message Queue"=w56) -> ("dup error in"=w57:errorcluster, "dup Message Queue"=w44:refnum<queue>)  [unwired: 8 in]
  }
  n161 = while {
    tunnel: w34 -> [w439]
    tunnel: [w441] -> w40
    shift-right: [w440] -> w35
    shift-left: w38 -> [w445]
    tunnel: [w438] -> w28
    tunnel: w27 -> [w438]
    tunnel: w13 -> [w437]
    shift-right: [w430] -> _
    shift-left: 50 ("Cycle") -> [w431]
    tunnel: [w429] -> w10
    tunnel: [w428] -> w9
    tunnel: w1 -> [w427]
    stop <- w444 stop-if-true
    # "Event Handling Loop"
    n162 = call "Dequeue Message.vi"("timeout in ms (-1)"=50, "Message Queue"=w437) -> ("error out"=w432:errorcluster, "Message Data"=w435:variant, "Message"=w436:string, "dup Message Queue"=w433:refnum<queue>)  [unwired: 6 in]
    n163 = Flush Queue(queue=w433, error in (no error)=w432) -> (queue out=w428:refnum<queue>)  [unwired: 2 out]
    n164 = case "Display Update" shown="\"Update\"" w436 {
      tunnel: w435 -> [_ w453]
      tunnel: w431 -> [w446 _]
      tunnel: [w446 w450] -> w430
      frame "False", Default {
      }
      frame "Update" {
        n165 = Variant To Data(type=T14 {"URL"="", "Cycle"=0, "Updating"=FALSE, "Tag Data"=[]} ("OPC Display Cluster"), Variant=w453) -> (data=w452:T14)  [unwired: 1 in, 1 out]
        n166 = Unbundle By Name(w452) -> ("URL"=→"server endpoint URL":string, "Cycle"=w450:i32, "Updating"=→"Updating":bool, "Tag Data"=→"Tag Data 2":T1[])
      }
    }
    n167 = event shown="[2] \"Exit\": Value Change" {
      selector: w445 -> [_ _ _ _ _ _]
      dyn-events: [_ _ _ _ _ _] -> w440
      timeout: w431 -> [_ _ _ _ _ _]
      tunnel: [_ _ TRUE ("Discard?") TRUE ("Discard?") _ _] -> w444
      tunnel: w439 -> [w454 w457 w463 w469 w474 w484]
      tunnel: [_ w455 w468 _ w476 _] -> w442
      tunnel: [w454 w456 w466 w469 w475 w484] -> w443
      tunnel: w427 -> [_ _ w461 _ _ _]
      event Timeout {
        n168 = event-data() -> ()  [unwired: 1 in, 1 out]
      }
      event Panel Close? {
        w458 = TRUE  # Priority Message
        n169 = event-data() -> ()  [unwired: 1 in, 1 out]
        n170 = call-poly "Enqueue Message.vi"("Priority Message? (F)"=w458, "Message"="Confirm Quit", "Message Queue"=w457) -> ("error out"=w455:errorcluster, "dup Message Queue"=w456:refnum<queue>)  [unwired: 7 in]
        n171 = event-data("Discard?"=TRUE) -> ()  [unwired: 1 in, 1 out]
      }
      event "Exit": Value Change {
        w464 = TRUE  # Priority Message
        # "The UI Message Loop handles sending the Exit message to other loops."
        n172 = event-data() -> ()  [unwired: 1 in, 1 out]
        n173 = call "Generate Temporary Report.vi"("Line of Events"=string[] ["Exit Clicked"], "Module Name"=w461) -> ()  [unwired: 9 in, 1 out]
        n174 = call-poly "Enqueue Message.vi"("Priority Message? (F)"=w464, "Message"="Exit", "Message Queue"=w463) -> ("error out"=w468:errorcluster, "dup Message Queue"=w466:refnum<queue>)  [unwired: 7 in]
      }
      event User Event {
        # "The Message Handling Loop processed an \"Exit\" message, which fired this event to stop the Event Handling Loop."
        n175 = event-data() -> ()  [unwired: 1 in, 1 out]
        n176 = local write "Status"("Exit" ("Exit String")) -> ()
      }
      event "Settings Button": Mouse Down {
        # "Allow debugging during run with a ctrl click"
        n177 = event-data() -> ("PlatMods"=w473:T15)  [unwired: 1 in]
        n178 = Unbundle By Name(w473) -> ("Ctrl"=w472:bool)
        n179 = case shown="False" w472 {
          tunnel: [w480 w481] -> w476
          tunnel: [w479 w482] -> w475
          tunnel: w474 -> [w478 w482]
          frame False {
            n180 = call-poly "Enqueue Message.vi"("Message"="Launch Settings Dialog", "Message Queue"=w478) -> ("error out"=w480:errorcluster, "dup Message Queue"=w479:refnum<queue>)  [unwired: 8 in]
          }
          frame True {
            n181 = property class="VI"("BDWin.Open"=TRUE ("Block Diagram Window:Open")) -> (error out=w481:errorcluster)  [unwired: 2 in, 1 out]
          }
        }
      }
      event Key Down {
        n182 = event-data() -> ("ScanCode"=→"ScanCode":i16)  [unwired: 1 in]
      }
    }
    n183 = call "Error Handler - Event Handling Loop.vi"("error in (no error)"=w442, "Message Queue"=w443) -> ("dup error in"=w441:errorcluster, "dup Message Queue"=w429:refnum<queue>)  [unwired: 8 in]
  }
  n184 = call "Main Loop.vi"("error in (no error)"=w16, "Chart Notifier"=w17, "Message Queues"=w18) -> ("error out"=w15:errorcluster)  [unwired: 8 in]
  n185 = Release Queue(queue=w9) -> ()  [unwired: 2 in, 3 out]
  n186 = Close Reference(reference=w28) -> ()  [unwired: 1 in, 1 out]
  n187 = Release Queue(queue=w10) -> ()  [unwired: 2 in, 3 out]
  n188 = Unregister For Events(event registration refnum=w35, error in=w40) -> (error out=w36:errorcluster)
  n189 = Merge Errors(w36, w41, w16, w15) -> (w39:errorcluster)
  n190 = Release Queue(queue=w8) -> ()  [unwired: 2 in, 3 out]
  n191 = call "Destroy User Event - Stop.vi"("error in (no error)"=w39, "User Event - Stop"=w37) -> ("error out"=w21:errorcluster)  [unwired: 9 in]
  n192 = flat-sequence {
    tunnel: w21 -> [_]
    frame #0 {
      n193 = invoke class="VI" method="FP.Close"() -> ()  [unwired: 3 in, 3 out]
    }
  }
